vi "PlateReaderTest.vi"() -> ()   [LabVIEW 2014]
uses:
  EventHandleInstrumentStatusChangedData.ctl
  EventHandleErrorReportData.ctl
  EventHandleCommandCompletedData.ctl
  C:/Program Files (x86)/Molecular Devices/SoftMax Pro 6.5.1 Automation SDK/SoftMaxPro.AutomationClient.dll
  Program Files (x86)/Molecular Devices/SoftMax Pro 6.5.1 Automation SDK/SoftMaxPro.AutomationClient.dll
  PlateReaderGlobal.vi
panel:
  in  "stop":bool
  out "Status":string
  out "ErrorReportQueue":T1[](array[typedef])
  out "CommandCompleteQueue":T2[](array[typedef])
  out "GetDataCopy":i32
  out "CommandCompleted":T2
  out "ErrorReport":T1
  out "InstrumentStatusChanged":T3
  out "StartRead":i32
  out "Initialize":bool
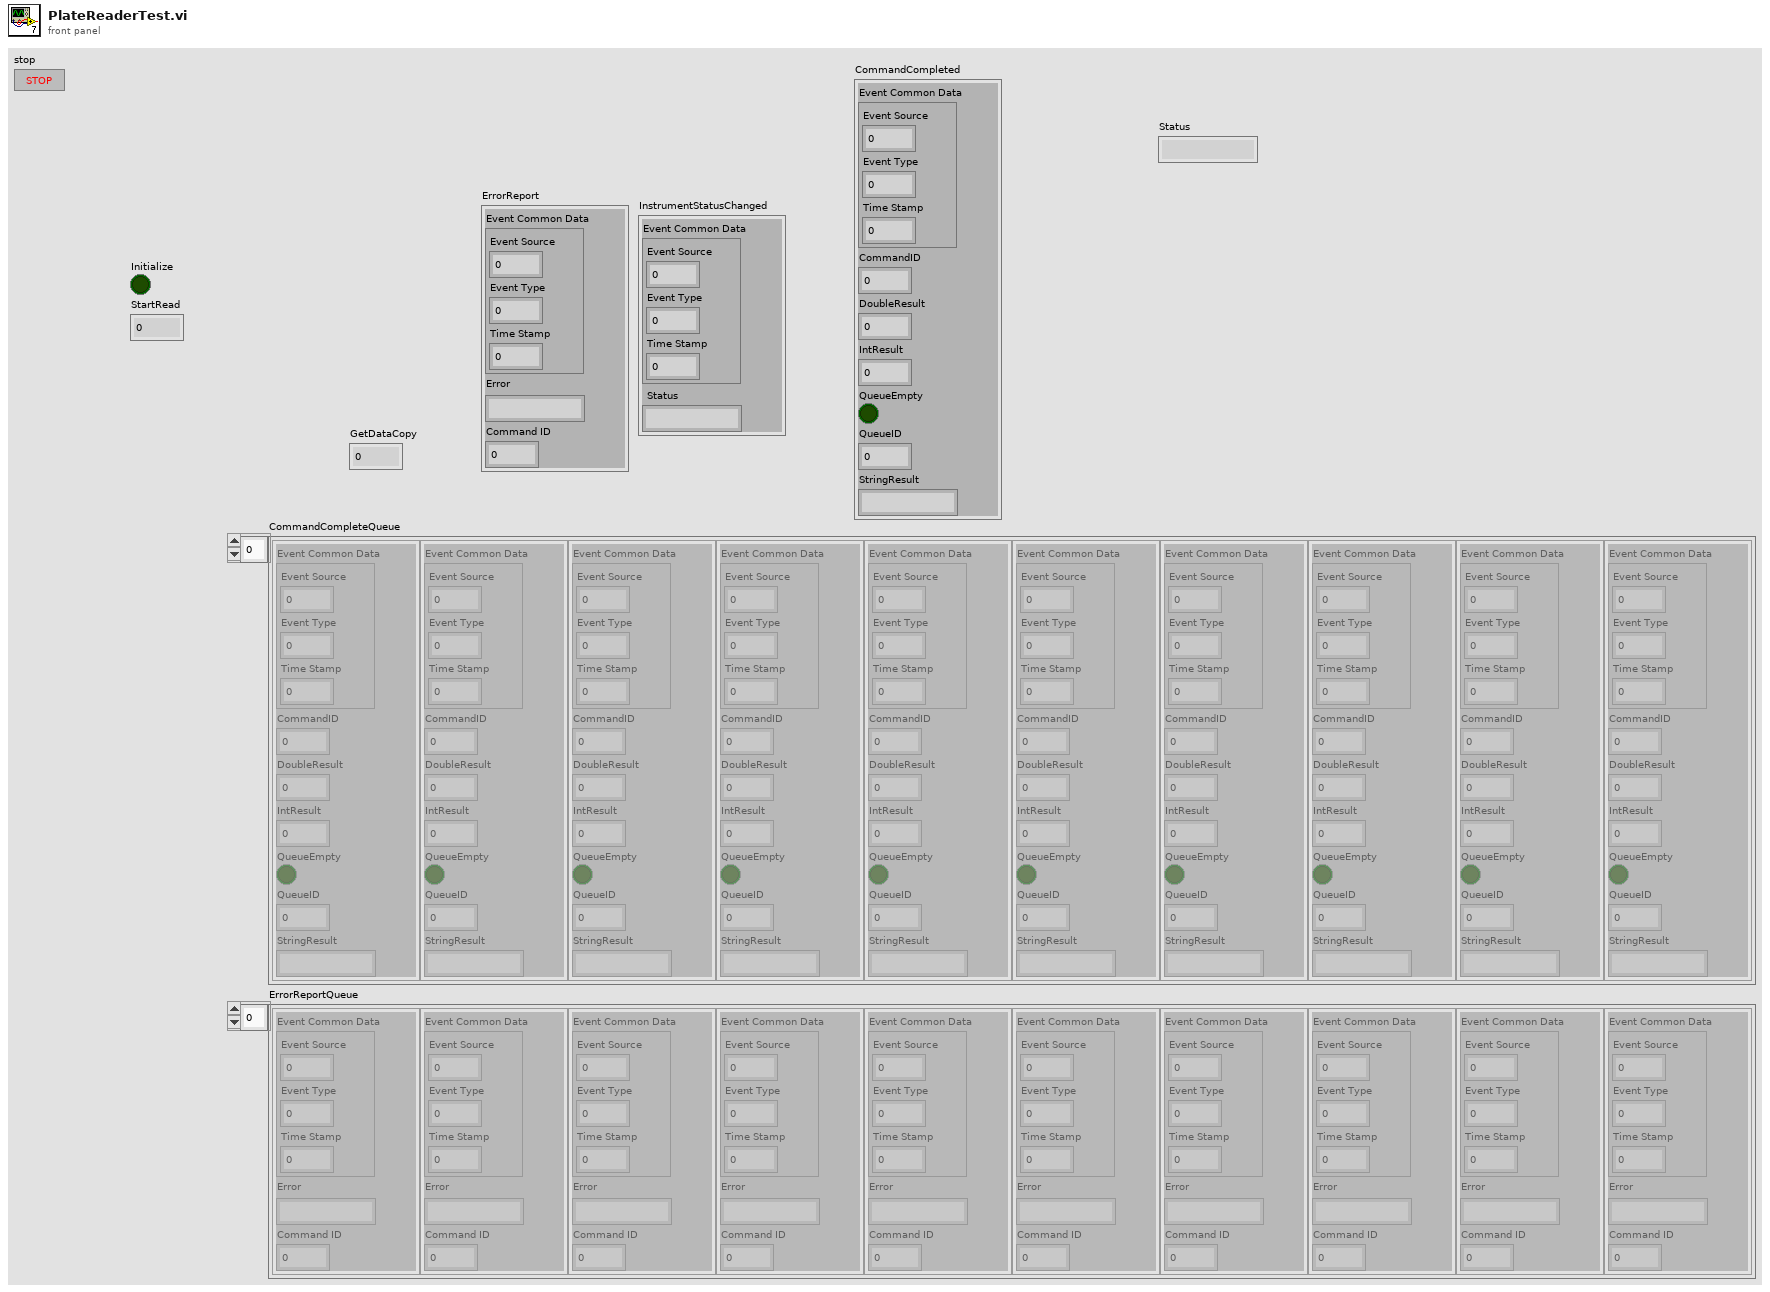
[diagram p1: front panel]
types:
  T1 = typedef "EventHandleErrorReportData.ctl" = cluster{"Event Common Data":cluster{"Event Source":i32, "Event Type":u32, "Time Stamp":u32}, "Error":string, "Command ID":i32}
  T2 = typedef "EventHandleCommandCompletedData.ctl" = cluster{"Event Common Data":cluster{"Event Source":i32, "Event Type":u32, "Time Stamp":u32}, "CommandID":i32, "DoubleResult":dbl, "IntResult":i32, "QueueEmpty":bool, "QueueID":i32, "StringResult":string}
  T3 = typedef "EventHandleInstrumentStatusChangedData.ctl" = cluster{"Event Common Data":cluster{"Event Source":i32, "Event Type":u32, "Time Stamp":u32}, "Status":string}
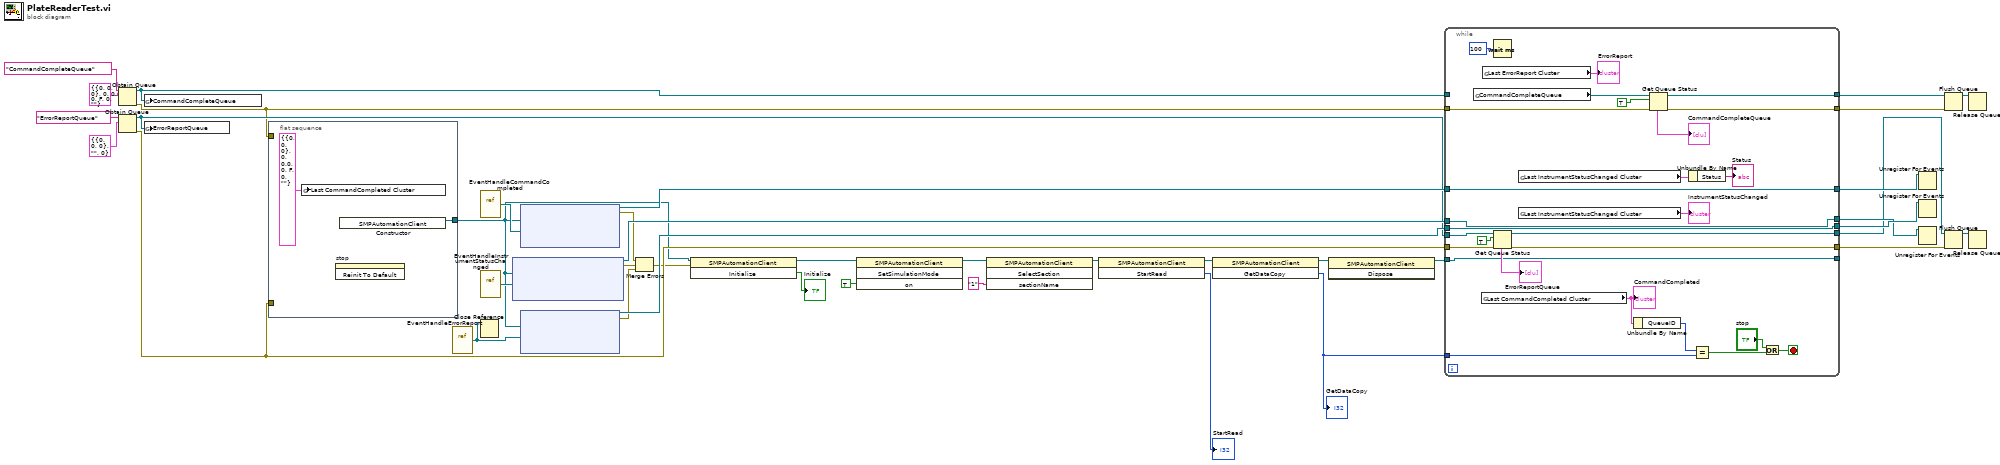
[diagram p0: block diagram]
diagram:
  n1 = Obtain Queue(name (unnamed)="CommandCompleteQueue", element data type=T2 {"Event Common Data"={"Event Source"=0, "Event Type"=0, "Time Stamp"=0}, "CommandID"=0, "DoubleResult"=0.0, "IntResult"=0, "QueueEmpty"=FALSE, "QueueID"=0, "StringResult"=""} ("Event Data Cluster")) -> (queue out=w19:refnum<queue>, error out=w14:errorcluster)  [unwired: 3 in, 1 out]
  n2 = Obtain Queue(name (unnamed)="ErrorReportQueue", element data type=T1 {"Event Common Data"={"Event Source"=0, "Event Type"=0, "Time Stamp"=0}, "Error"="", "Command ID"=0} ("ErrorReport Data")) -> (queue out=w17:refnum<queue>, error out=w15:errorcluster)  [unwired: 3 in, 1 out]
  n3 = global write "PlateReaderGlobal.vi" "CommandCompleteQueue"(w19) -> ()
  n4 = global write "PlateReaderGlobal.vi" "ErrorReportQueue"(w17) -> ()
  n5 = flat-sequence {
    tunnel: [w41] -> w12
    tunnel: w15 -> [_]
    tunnel: w14 -> [_]
    frame #0 {
      n6 = global write "PlateReaderGlobal.vi" "Last CommandCompleted Cluster"(T2 {"Event Common Data"={"Event Source"=0, "Event Type"=0, "Time Stamp"=0}, "CommandID"=0, "DoubleResult"=0.0, "IntResult"=0, "QueueEmpty"=FALSE, "QueueID"=0, "StringResult"=""} ("Last CommandCompleted Cluster")) -> ()
      n7 = invoke on="stop" class="Bool (strict)" method="Reinit To Default"() -> ()  [unwired: 3 in, 3 out]
      n8 = constructor class="SMPAutomationClient"() -> (reference out=w41:refnum<k24>)  [unwired: 3 in, 2 out]
    }
  }
  n9 = vi-ref "EventHandleErrorReport.vi"() -> ("vi reference"=w28:refnum<vi>)
  n10 = vi-ref "EventHandleCommandCompleted.vi"() -> ("vi reference"=w33:refnum<vi>)
  n11 = vi-ref "EventHandleInstrumentStatusChanged.vi"() -> ("vi reference"=w32:refnum<vi>)
  n12 = Close Reference(reference=w28) -> ()  [unwired: 1 in, 1 out]
  n13 = node(w12, w32) -> (w34:refnum<k27>, w30:errorcluster)  [unwired: 3 in]
  n14 = node(w12, w33) -> (w38:refnum<k27>, w31:errorcluster)  [unwired: 3 in]
  n15 = node(w12, w28) -> (w36:refnum<k27>, w29:errorcluster)  [unwired: 3 in]
  n16 = Merge Errors(w31, w30, w29) -> (w13:errorcluster)
  n17 = invoke class="SMPAutomationClient" method="Initialize"(reference=w12, error in=w13) -> (reference out=w3:refnum<k24>, "Initialize"=→"Initialize":bool)  [unwired: 1 in, 1 out]
  n18 = invoke class="SMPAutomationClient" method="SetSimulationMode"(reference=w3, "on"=TRUE) -> (reference out=w8:refnum<k24>)  [unwired: 2 in, 3 out]
  n19 = invoke class="SMPAutomationClient" method="SelectSection"(reference=w8, "sectionName"="1") -> (reference out=w7:refnum<k24>)  [unwired: 2 in, 3 out]
  n20 = invoke class="SMPAutomationClient" method="StartRead"(reference=w7) -> (reference out=w5:refnum<k24>, "StartRead"=→"StartRead":i32)  [unwired: 2 in, 1 out]
  n21 = invoke class="SMPAutomationClient" method="GetDataCopy"(reference=w5) -> (reference out=w2:refnum<k24>, "GetDataCopy"=w4:i32)  [unwired: 2 in, 1 out]
  "GetDataCopy" <- w4
  n22 = invoke class="SMPAutomationClient" method="Dispose"(reference=w2) -> (reference out=w1:refnum<k24>)  [unwired: 2 in, 2 out]
  n23 = while {
    tunnel: [w68] -> w39
    tunnel: w38 -> [w68]
    tunnel: w1 -> [w42]
    tunnel: [w67] -> w37
    tunnel: w36 -> [w67]
    tunnel: [w66] -> w35
    tunnel: w34 -> [w66]
    tunnel: w14 -> [w59]
    tunnel: [w58] -> w21
    tunnel: w15 -> [w57]
    tunnel: [w56] -> w20
    tunnel: w19 -> [_]
    tunnel: [w55] -> w18
    tunnel: w17 -> [w54]
    tunnel: [w53] -> w16
    tunnel: w4 -> [w47]
    tunnel: [w42] -> _
    stop <- w44 stop-if-true
    n24 = global read "PlateReaderGlobal.vi" "CommandCompleteQueue"() -> (w51:refnum<queue>)
    n25 = global read "PlateReaderGlobal.vi" "Last CommandCompleted Cluster"() -> (w48:T2)
    "CommandCompleted" <- w48
    n26 = global read "PlateReaderGlobal.vi" "Last ErrorReport Cluster"() -> (→"ErrorReport":T1)
    n27 = Wait (ms)(milliseconds to wait=u32 100) -> ()  [unwired: 1 out]
    n28 = Get Queue Status(queue=w54, return elements? (F)=TRUE, error in (no error)=w57) -> (queue out=w53:refnum<queue>, error out=w56:errorcluster, elements=→"ErrorReportQueue":T1[])  [unwired: 5 out]
    n29 = global read "PlateReaderGlobal.vi" "Last InstrumentStatusChanged Cluster"() -> (w60:T3)
    n30 = global read "PlateReaderGlobal.vi" "Last InstrumentStatusChanged Cluster"() -> (→"InstrumentStatusChanged":T3)
    n31 = Unbundle By Name(w48) -> ("QueueID"=w46:i32)
    n32 = Get Queue Status(queue=w51, return elements? (F)=TRUE, error in (no error)=w59) -> (queue out=w55:refnum<queue>, error out=w58:errorcluster, elements=→"CommandCompleteQueue":T2[])  [unwired: 5 out]
    n33 = Unbundle By Name(w60) -> ("Status"=→"Status":string)
    n34 = Equal?(x=w46, y=w47) -> (x = y?=w45:bool)
    n35 = Or(x="stop", y=w45) -> (x .or. y?=w44:bool)
  }
  n36 = Unregister For Events(event registration refnum=w39) -> ()  [unwired: 1 in, 1 out]
  n37 = Unregister For Events(event registration refnum=w37) -> ()  [unwired: 1 in, 1 out]
  n38 = Unregister For Events(event registration refnum=w35) -> ()  [unwired: 1 in, 1 out]
  n39 = Flush Queue(queue=w18, error in (no error)=w21) -> (queue out=w23:refnum<queue>)  [unwired: 2 out]
  n40 = Flush Queue(queue=w16, error in (no error)=w20) -> (queue out=w22:refnum<queue>)  [unwired: 2 out]
  n41 = Release Queue(queue=w23) -> ()  [unwired: 2 in, 3 out]
  n42 = Release Queue(queue=w22) -> ()  [unwired: 2 in, 3 out]
